vi "_TangoStateColor.vi"(1 "State":u32) -> (0 "State Color":u32(colorbox)=16448250)   [LabVIEW 2014, in "tango.lvlib"]
uses:
  tango.lvlib
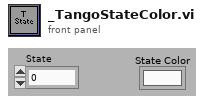
[diagram p1: front panel]
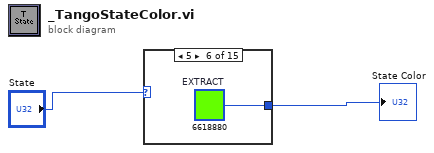
[diagram p0: block diagram]
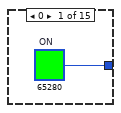
[diagram p2: hidden frame]
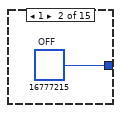
[diagram p3: hidden frame]
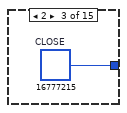
[diagram p4: hidden frame]
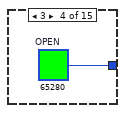
[diagram p5: hidden frame]
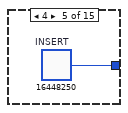
[diagram p6: hidden frame]
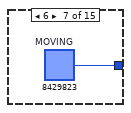
[diagram p7: hidden frame]
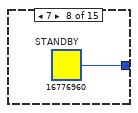
[diagram p8: hidden frame]
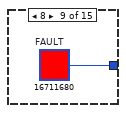
[diagram p9: hidden frame]
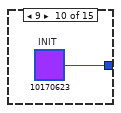
[diagram p10: hidden frame]
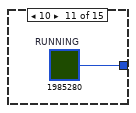
[diagram p11: hidden frame]
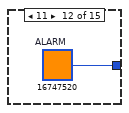
[diagram p12: hidden frame]
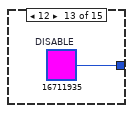
[diagram p13: hidden frame]
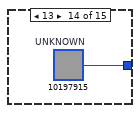
[diagram p14: hidden frame]
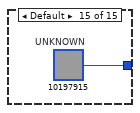
[diagram p15: hidden frame]
diagram:
  n1 = case shown="5" "State" {
    tunnel: [w3 w4 w5 w6 w7 w8 w9 w10 w11 w12 w13 w14 w15 w16 w17] -> w2
    frame 0 {
      w3 = u32 65280  # ON
    }
    frame 1 {
      w4 = u32 16777215  # OFF
    }
    frame 2 {
      w5 = u32 16777215  # CLOSE
    }
    frame 3 {
      w6 = u32 65280  # OPEN
    }
    frame 4 {
      w7 = u32 16448250  # INSERT
    }
    frame 5 {
      w8 = u32 6618880  # EXTRACT
    }
    frame 6 {
      w9 = u32 8429823  # MOVING
    }
    frame 7 {
      w10 = u32 16776960  # STANDBY
    }
    frame 8 {
      w11 = u32 16711680  # FAULT
    }
    frame 9 {
      w12 = u32 10170623  # INIT
    }
    frame 10 {
      w13 = u32 1985280  # RUNNING
    }
    frame 11 {
      w14 = u32 16747520  # ALARM
    }
    frame 12 {
      w15 = u32 16711935  # DISABLE
    }
    frame 13 {
      w16 = u32 10197915  # UNKNOWN
    }
    frame Default {
      w17 = u32 10197915  # UNKNOWN
    }
  }
  "State Color" <- w2
